vi "ziModGetZoomFFTData.vi"(8 "Error In":errorcluster, 10 "ModResults":T2, 11 "ModHandle In":T5 {"ModHandle" format="0x%08x"; "Conn" format="0x%08x"}) -> (0 "Error Out":errorcluster, 2 "SpectrumWaveArray":T1[](array[typedef]) {"overlap" format="%f"; "nenbw" format="%f"; "center" format="%f"; "resolution" format="%f"; "aliasingReject" format="%f"; "rate" format="%f"; "bandwidth" format="%f"; "window" format="%f"; "flags" format="%f"; "sampleFormat" format="%f"; "spectrumMode" format="%f"; "sampleCount" format="%f"; "timestamp" format="%f"}, 3 "ModHandle Out":T5 {"ModHandle" format="0x%08x"; "Conn" format="0x%08x"})   [LabVIEW 2009, in "Zurich Instruments LabOne.lvlib"]
doc: "Use this vi to get SpectrumData from a ModResult returned from ziModGetNextNode.vi. It returns an array of SpectrumData."
uses:
  <instrlib>/Zurich Instruments LabOne/Zurich Instruments LabOne.lvlib
  <instrlib>/Zurich Instruments LabOne/Public/Modules/ziTypeModHandle.ctl
  <instrlib>/Zurich Instruments LabOne/Public/Modules/ziTypeModResults.ctl
  <instrlib>/Zurich Instruments LabOne/Public/Data/ziTypePollType.ctl
  <instrlib>/Zurich Instruments LabOne/Public/Modules/ziTypeModGenericHeader.ctl
  <instrlib>/Zurich Instruments LabOne/Public/Modules/ziTypeModSpectrumWave.ctl
  <instrlib>/Zurich Instruments LabOne/Private/ziLV32.dll
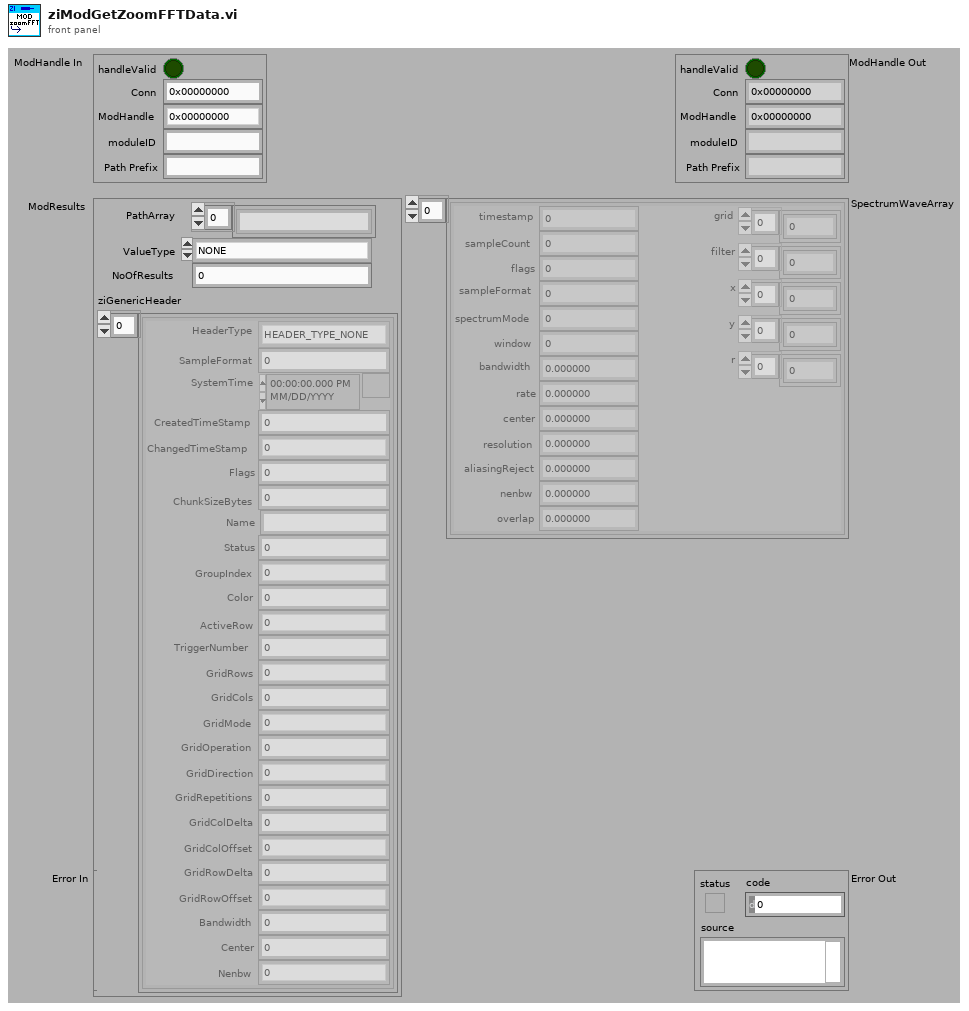
[diagram p1: front panel]
types:
  T1 = typedef "Zurich Instruments LabOne.lvlib/ziTypeModSpectrumWave.ctl" = cluster{"timestamp":u64, "sampleCount":u64, "flags":u8, "sampleFormat":u8, "spectrumMode":u8, "window":u8, "bandwidth":dbl, "rate":dbl, "center":dbl, "resolution":dbl, "aliasingReject":dbl, "nenbw":dbl, "overlap":dbl, "grid":dbl[], "filter":dbl[], "x":dbl[], "y":dbl[], "r":dbl[]}
  T2 = typedef "Zurich Instruments LabOne.lvlib/ziTypeModResults.ctl" = cluster{"PathArray":string[], "ValueType":T3, "NoOfResults":u64, "ziGenericHeader":T4[]}
  T3 = typedef "Zurich Instruments LabOne.lvlib/ziTypePollType.ctl" = enum16{"NONE", "DOUBLE_DATA", "INTEGER_DATA", "DEMOD_SAMPLE", "SCOPE_WAVE_HF2", "AUXIN_SAMPLE", "DIO_SAMPLE", "BYTE_ARRAY", "PWA_WAVE", "9", "10", "11", "12", "13", "14", "15", "TREE_CHANGE_DEPRI", "17", "ERROR", "19", "20", "21", "22", "23", "24", "25", "26", "27", "28", "29", "30", "31", "DOUBLE_DATA_TS", "INTEGER_DATA_TS", "34", "SCOPE_WAVE", "SCOPE_WAVE_EX", "37", "BYTE_ARRAY_TS", "39", "40", "41", "42", "43", "44", "45", "CNT_DATA", "47", "TREE_CHANGE", "49", "50", "51", "52", "53", "54", "55", "56", "57", "58", "59", "60", "61", "62", "63", "SWEEPER_DATA", "SPECTRUM_DATA", "ADVISOR_DATA", "VECTOR_DATA", "IMP_DATA"}
  T4 = typedef "Zurich Instruments LabOne.lvlib/ziTypeModGenericHeader.ctl" = cluster{"HeaderType":enum8{"HEADER_TYPE_NONE", "HEADER_TYPE_SWTRIGGER", "HEADER_TYPE_SWEEPER"}, "SampleFormat":u8, "SystemTime":timestamp, "CreatedTimeStamp":u64, "ChangedTimeStamp":u64, "Flags":u32, "ChunkSizeBytes":u64, "Name":string, "Status":u32, "GroupIndex":u32, "Color":u32, "ActiveRow":u32, "TriggerNumber":u64, "GridRows":u32, "GridCols":u32, "GridMode":u32, "GridOperation":u32, "GridDirection":u32, "GridRepetitions":u32, "GridColDelta":dbl, "GridColOffset":dbl, "GridRowDelta":dbl, "GridRowOffset":dbl, "Bandwidth":dbl, "Center":dbl, "Nenbw":dbl}
  T5 = typedef "Zurich Instruments LabOne.lvlib/ziTypeModHandle.ctl" = cluster{"handleValid":bool, "Conn":u64, "ModHandle":u64, "moduleID":string, "Path Prefix":string}
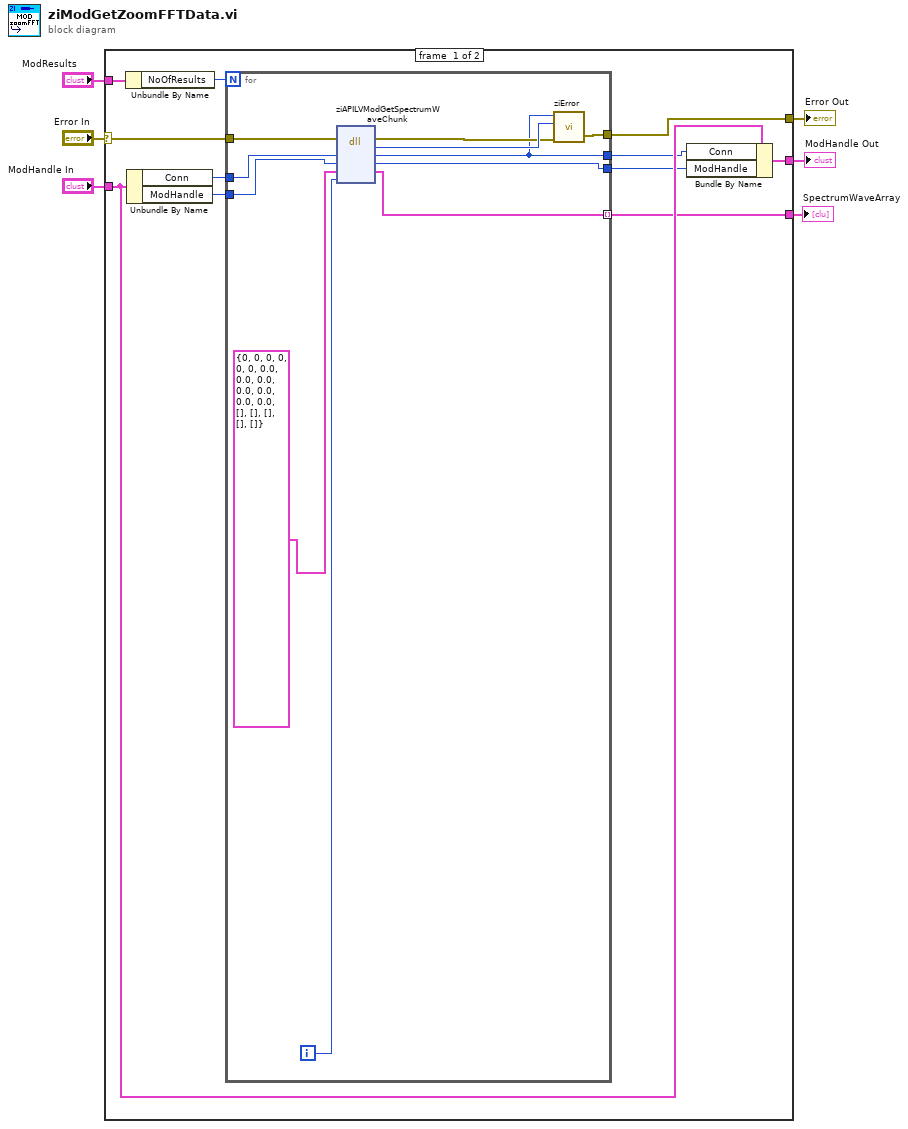
[diagram p0: block diagram]
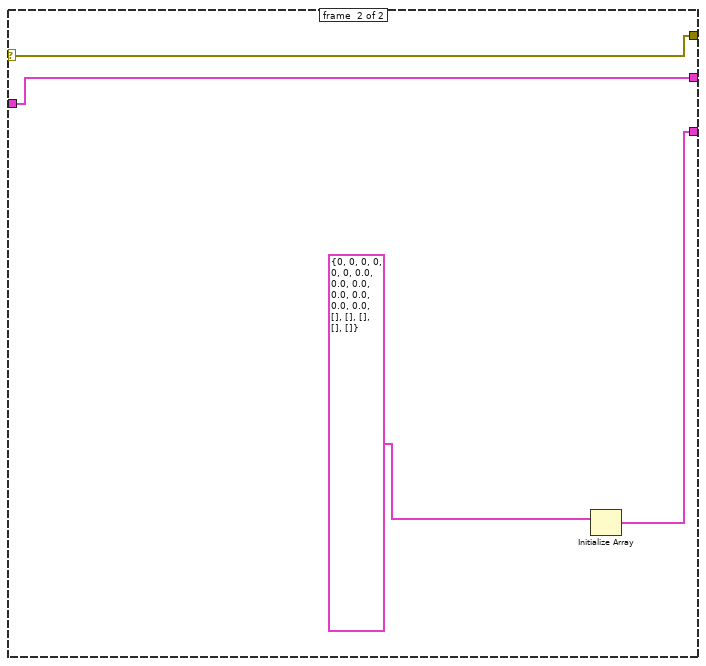
[diagram p2: hidden frame]
diagram:
  n1 = case shown="No Error" "Error In" {
    selector: "Error In" -> [w8 w31]
    tunnel: [w9 w31] -> w2
    tunnel: [w16 w32] -> w5
    tunnel: "ModHandle In" -> [w17 w32]
    tunnel: "ModResults" -> [w13 _]
    tunnel: [w7 w30] -> w1
    frame #0 {
      n2 = Unbundle By Name(w13) -> ("NoOfResults"=w12:u64)
      n3 = Unbundle By Name(w17) -> ("Conn"=w15:u64, "ModHandle"=w14:u64)
      n4 = for {
        N: w12 -> [_]
        tunnel: [w18] -> w11
        tunnel: [w28] -> w10
        tunnel: w15 -> [w27]
        tunnel: w14 -> [w26]
        tunnel: [w24] -> w9
        tunnel: w8 -> [w21]
        tunnel: [w20] -> w7 mode=indexing
        i -> [w25]
        n5 = dll-call lib="C:/Program Files (x86)/National Instruments/LabVIEW 2009/instr.lib/Zurich Instruments LabOne/Private/ziLV*.*" fn="ziAPILVModGetSpectrumWaveChunk"(error in=w21, "Conn"=w27, "ModHandle"=w26, "SweeperWave"=T1 {"timestamp"=0, "sampleCount"=0, "flags"=0, "sampleFormat"=0, "spectrumMode"=0, "window"=0, "bandwidth"=0.0, "rate"=0.0, "center"=0.0, "resolution"=0.0, "aliasingReject"=0.0, "nenbw"=0.0, "overlap"=0.0, "grid"=[], "filter"=[], "x"=[], "y"=[], "r"=[]} ("ziModSpectrumWave"), "chunk_idx"=w25) -> (error out=w22:errorcluster, "return type"=w23:u32, "Conn"=w18:u64, "ModHandle"=w28:u64, "SweeperWave"=w20:T1)  [unwired: 3 in, 1 out]
        n6 = call <instrlib>:"ziError.vi"("Conn"=w18, "ziErrorCode"=w23, "Error In"=w22) -> ("Error Out"=w24:errorcluster)  [unwired: 2 in, 1 out]
      }
      n7 = Bundle By Name(cluster=w17, "Conn"=w11, "ModHandle"=w10) -> (w16:T5)
    }
    frame #1 {
      n8 = Initialize Array(T1 {"timestamp"=0, "sampleCount"=0, "flags"=0, "sampleFormat"=0, "spectrumMode"=0, "window"=0, "bandwidth"=0.0, "rate"=0.0, "center"=0.0, "resolution"=0.0, "aliasingReject"=0.0, "nenbw"=0.0, "overlap"=0.0, "grid"=[], "filter"=[], "x"=[], "y"=[], "r"=[]} ("ziModSpectrumWave")) -> (w30:T1[])  [unwired: 1 in]
    }
  }
  "Error Out" <- w2
  "ModHandle Out" <- w5
  "SpectrumWaveArray" <- w1
